vi "Variant to Alarm Status.vi"(8 "error in":errorcluster, 11 "value":variant) -> (0 "error out":errorcluster, 1 "Message":string, 2 "Severity":T1, 3 "value out":variant, 5 "Status":T2(ring))   [LabVIEW 2020, in "Value.lvlib"]
uses:
  Value.lvlib
  Alarm Severity.ctl
  Alarm Status.ctl
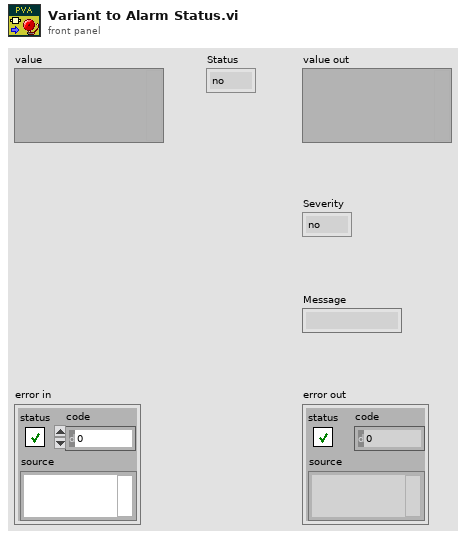
[diagram p1: front panel]
types:
  T1 = typedef "Value.lvlib/Alarm Severity.ctl" = enum32{"no", "minor", "major", "record", "invalid", "undefined", ""}
  T2 = enum32{"no", "device", "driver", "record", "db", "conf", "undefined", "client"}
  T3 = typedef "Value.lvlib/Alarm Status.ctl" = cluster{"Severity":T1, "Status":enum32{"no", "device", "driver", "record", "db", "conf", "undefined", "client"}, "Message":string}
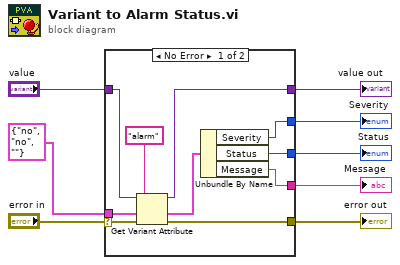
[diagram p0: block diagram]
diagram:
  n1 = case shown="No Error" "error in" {
    selector: "error in" -> [w17 w20]
    tunnel: [w11 w20] -> w8
    tunnel: "value" -> [w18 w19]
    tunnel: [w9 w19] -> w5
    tunnel: T3 {"Severity"=enum."no", "Status"=enum."no", "Message"=""} ("Alarm") -> [w15 _]
    tunnel: [w13 _] -> w1
    tunnel: [w12 _] -> w3
    tunnel: [w10 _] -> w2
    frame No Error {
      n2 = Get Variant Attribute(Variant=w18, name="alarm", default value (empty Variant)=w15, error in=w17) -> (duplicate Variant=w9:variant, value=w14:T3, error out=w11:errorcluster)  [unwired: 1 out]
      n3 = Unbundle By Name(w14) -> ("Severity"=w13:T1, "Status"=w12:T2, "Message"=w10:string)
    }
    frame Error {
    }
  }
  "error out" <- w8
  "value out" <- w5
  "Status" <- w3
  "Message" <- w2
  "Severity" <- w1
